vi "RegisterSALEvents.vi"(8 "error in (no error)":errorcluster, 10 "Event Registration Refnum In":refnum<event-registration>, 11 "SAL in":refnum<class "SAL.lvclass">) -> (0 "error out":errorcluster, 2 "Event Registration Refnum Out":refnum<event-registration>, 3 "SAL out":refnum<class "SAL.lvclass">)   [LabVIEW 2016, in "SAL.lvclass"]
uses:
  SAL.lvclass
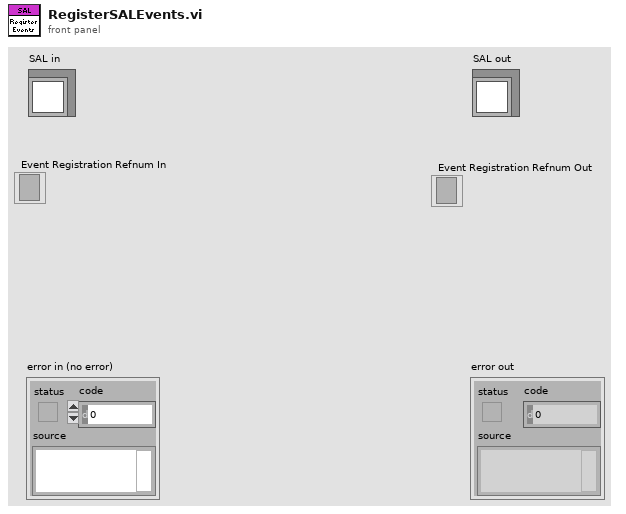
[diagram p1: front panel]
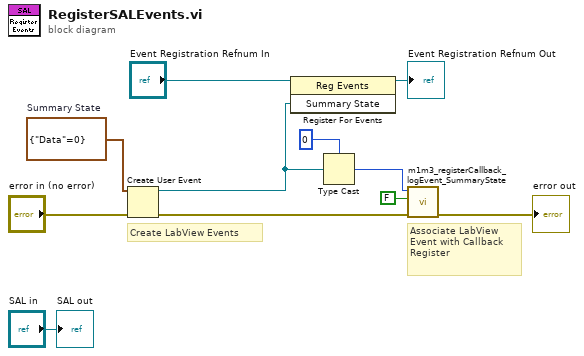
[diagram p0: block diagram]
diagram:
  w7 = cluster{"Data":i32} {"Data"=0}  # Summary State
  # "Associate LabView\nEvent with Callback\nRegister"
  # "Create LabView Events"
  n1 = Create User Event(user event datatype=w7, error in="error in (no error)") -> (user event=w4:refnum<user-event>, error out=w10:errorcluster)
  n2 = register-events(reference="Event Registration Refnum In", w4) -> (reference out=→"Event Registration Refnum Out":refnum<event-registration>)  [unwired: 1 in, 1 out]
  n3 = Type Cast(type=0, x=w4) -> (*(type *) &x=w9:i32)
  n4 = call "m1m3_registerCallback_logEvent_SummaryState.vi"("error in (no error)"=w10, "skipOld"=FALSE, "handle"=w9) -> ("error out"=→"error out":errorcluster)  [unwired: 7 in, 1 out]
  "SAL out" <- "SAL in"
